vi "Get Current Temperature.vi"(0 "VISA resource name":refnum<visa-resource-name>, 11 "error in (no error)":errorcluster) -> (4 "VISA resource name out":refnum<visa-resource-name>, 8 "Current Temperature (C)":dbl, 15 "error out":errorcluster)   [LabVIEW 2023, in "ACM Visa Driver.lvlib"]
uses:
  ACM Visa Driver.lvlib
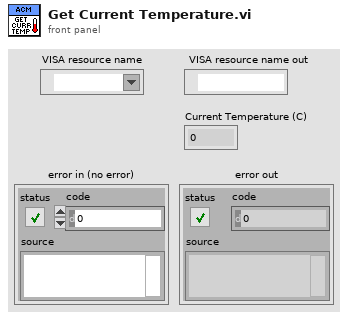
[diagram p1: front panel]
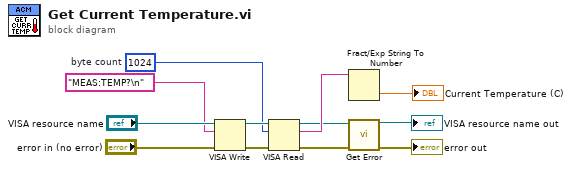
[diagram p0: block diagram]
diagram:
  w6 = u32 1024  # byte count
  n1 = VISA Write(VISA resource name="VISA resource name", write buffer="MEAS:TEMP?\n", error in (no error)="error in (no error)") -> (VISA resource name out=w7:refnum<visa-resource-name>, error out=w9:errorcluster)  [unwired: 1 out]
  n2 = VISA Read(VISA resource name=w7, byte count=w6, error in (no error)=w9) -> (VISA resource name out=w2:refnum<visa-resource-name>, read buffer=w5:string, error out=w8:errorcluster)  [unwired: 1 out]
  n3 = Fract/Exp String To Number(string=w5) -> (number=→"Current Temperature (C)":dbl)  [unwired: 3 in, 1 out]
  n4 = call "Get Error.vi"("VISA resource name"=w2, "error in (no error)"=w8) -> ("VISA resource name out"=→"VISA resource name out":refnum<visa-resource-name>, "error out"=→"error out":errorcluster)  [unwired: 12 in]
